vi "Path to Script.vi"(7 "Device Name":string, 8 "error in (no error)":errorcluster, 9 "Script Name":string, 10 "Path to script":string, 11 "pytoml file path":string) -> (0 "error out":errorcluster)   [LabVIEW 2020]
panel:
  out "return code":i32
  out "standard error":string
  out "standard output":string
  out "path":path
  out "result string":string
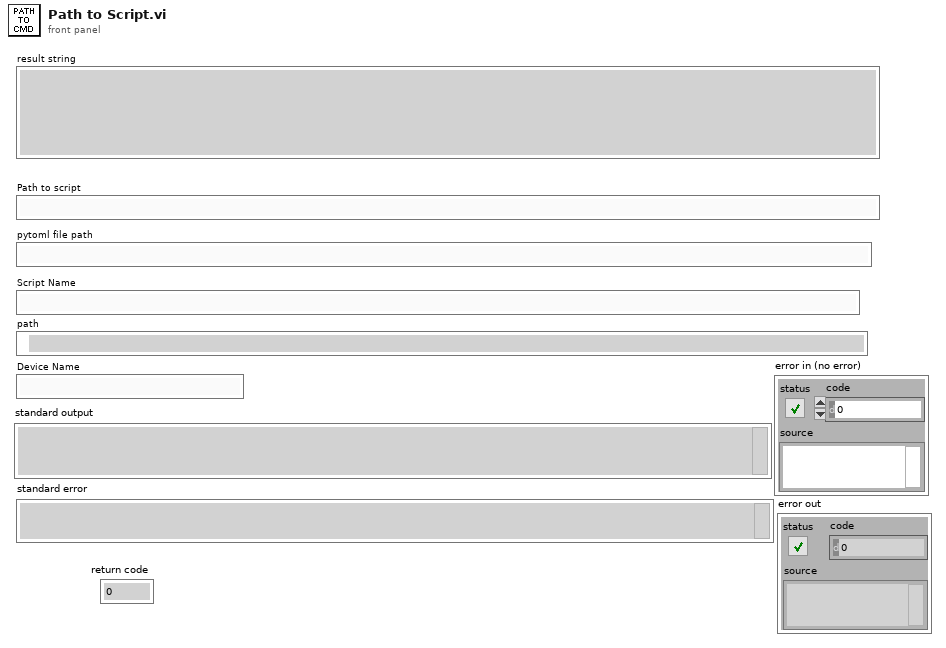
[diagram p1: front panel]
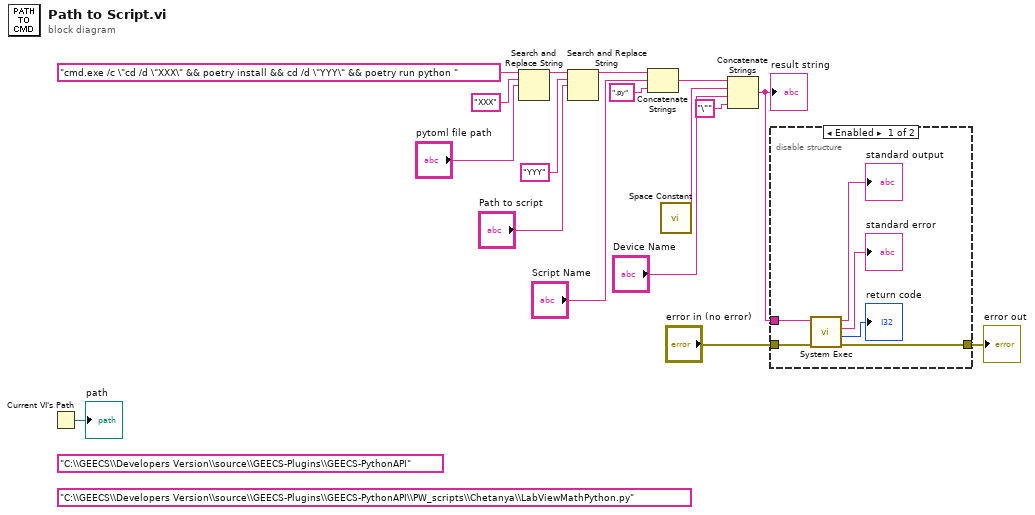
[diagram p0: block diagram]
diagram:
  (unwired) "C:\\GEECS\\Developers Version\\source\\GEECS-Plugins\\GEECS-PythonAPI\\PW_scripts\\Chetanya\\LabViewMathPython.py"
  (unwired) "C:\\GEECS\\Developers Version\\source\\GEECS-Plugins\\GEECS-PythonAPI" ("replace string (\"\")")
  n1 = Current VI's Path() -> (path=→"path":path)
  n2 = Search and Replace String(input string="cmd.exe /c \"cd /d \"XXX\" && poetry install && cd /d \"YYY\" && poetry run python ", search string="XXX" ("substring (\"\")"), replace string="pytoml file path") -> (result string=w15:string)  [unwired: 5 in, 3 out]
  n3 = Search and Replace String(input string=w15, search string="YYY", replace string="Path to script") -> (result string=w4:string)  [unwired: 5 in, 3 out]
  n4 = Concatenate Strings(w4, "Script Name", ".py" ("string")) -> (w3:string)
  n5 = call "Space Constant.vi"() -> ("String"=w10:string)
  n6 = Concatenate Strings(w3, w10, "Device Name", "\"" ("string")) -> (w6:string)
  "result string" <- w6
  n7 = disable-structure shown="Enabled" {
    disable-tunnel: w6 -> [w20 _]
    disable-tunnel: "error in (no error)" -> [w19 _]
    disable-tunnel: [w18 _] -> w1
    frame Enabled {
      n8 = call "System Exec.vi"("error in (no error)"=w19, "command line"=w20) -> ("error out"=w18:errorcluster, "return code"=→"return code":i32, "standard error"=→"standard error":string, "standard output"=→"standard output":string)  [unwired: 6 in]
    }
    frame Disabled {
    }
  }
  "error out" <- w1
